vi "parseAttributeType.vi"(8 "error in (no error)":errorcluster, 10 "XML in":string, 11 "AttributeReader in":refnum<class "XMLAttributeParser.lvclass">) -> (0 "error out":errorcluster, 2 "ParsedTypes":string[](array[string]), 3 "AttributeReader out":refnum<class "XMLAttributeParser.lvclass">)   [LabVIEW 2014, in "XML.lvlib" / "XMLAttributeParser.lvclass"]
doc: "This method finds anything in the open tag of the form (inside the square brackets) [AttributeType=], throws away the equals sign and parses the type.a"
uses:
  <userlib>/Common/XML/XMLAttributeParser/XMLAttributeParser.lvclass
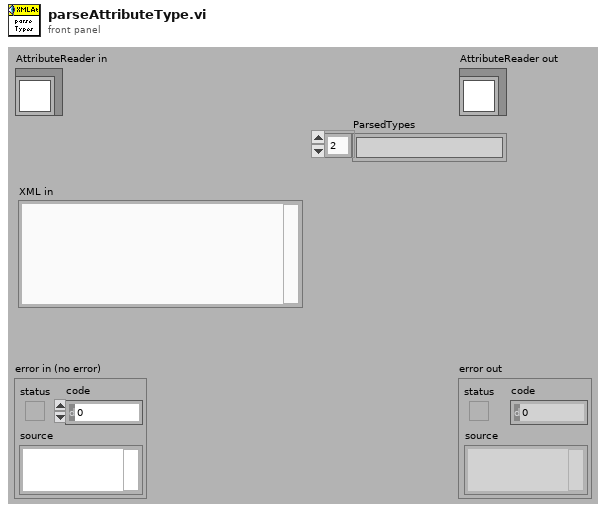
[diagram p1: front panel]
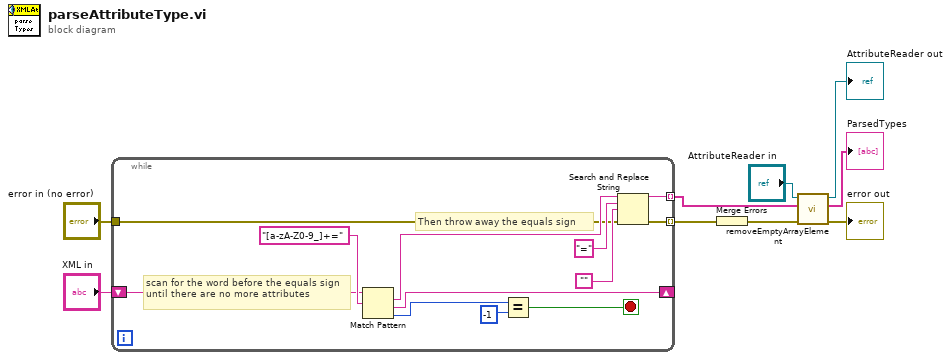
[diagram p0: block diagram]
diagram:
  n1 = while {
    shift-right: [w16] -> _
    shift-left: "XML in" -> [w18]
    tunnel: [w12] -> w6 mode=indexing
    tunnel: "error in (no error)" -> [w11]
    tunnel: [w10] -> w8 mode=indexing
    stop <- w17 stop-if-true
    # "Then throw away the equals sign"
    # "scan for the word before the equals sign until there are no more attributes"
    n2 = Match Pattern(string=w18, regular expression="[a-zA-Z0-9_]+=") -> (match substring=w13:string, after substring=w16:string, offset past match=w20:i32)  [unwired: 1 in, 1 out]
    n3 = Equal?(x=w20, y=-1) -> (x = y?=w17:bool)
    n4 = Search and Replace String(input string=w13, search string="=", replace string="", error in=w11) -> (result string=w12:string, error out=w10:errorcluster)  [unwired: 4 in, 2 out]
  }
  n5 = Merge Errors(w8) -> (w4:errorcluster)
  n6 = call <userlib>:"removeEmptyArrayElement.vi"("error in (no error)"=w4, "Array in"=w6, "AttributeReader in"="AttributeReader in") -> ("error out"=→"error out":errorcluster, "Array out"=→"ParsedTypes":string[], "AttributeReader out"=→"AttributeReader out":refnum<class "XMLAttributeParser.lvclass">)  [unwired: 6 in]
